vi "lsl get session id.vi"(8 "error in (no error)":errorcluster, 11 "streaminfo":T1) -> (0 "error out":errorcluster, 3 "session ID":string)   [LabVIEW 2016, in "Lab Streaming Layer.lvlib"]
doc: "extern LIBLSL_C_API const char *lsl_get_session_id(lsl_streaminfo info);"
uses:
  Lab Streaming Layer.lvlib
  liblsl-LabVIEW-master/liblsl-LabVIEW-master/lsl.dll
  Custom Controls/lsl_streaminfo.ctl
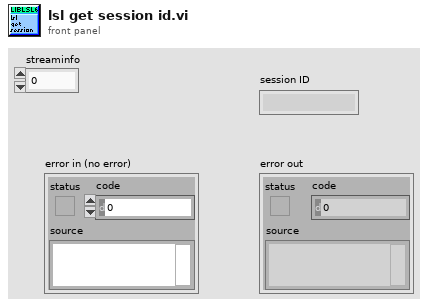
[diagram p1: front panel]
types:
  T1 = typedef "liblsl-LabVIEW.lvlib/lsl_streaminfo.ctl" = u64
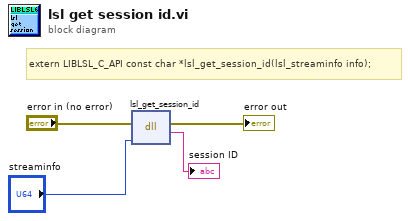
[diagram p0: block diagram]
diagram:
  # "extern LIBLSL_C_API const char *lsl_get_session_id(lsl_streaminfo info);"
  n1 = dll-call lib="E:/LabStreamingLayer/liblsl-LabVIEW-master/liblsl-LabVIEW-master/lsl.dll" fn="lsl_get_session_id"(error in="error in (no error)", "info"="streaminfo") -> (error out=→"error out":errorcluster, "return type"=→"session ID":string)  [unwired: 3 in, 1 out]
